vi "visa_close.vi"(2 "err_in":errorcluster, 4 "thcd_visa":refnum<visa-resource-name>) -> (0 "err_out":errorcluster)   [LabVIEW 2019]
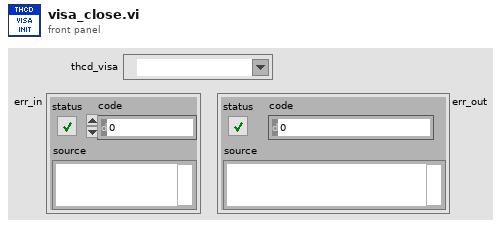
[diagram p1: front panel]
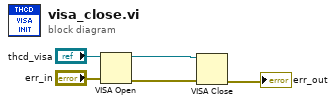
[diagram p0: block diagram]
diagram:
  n1 = VISA Open(error in (no error)="err_in", VISA resource name="thcd_visa") -> (VISA resource name=w1:refnum<visa-resource-name>, error out=w3:errorcluster)  [unwired: 3 in]
  n2 = VISA Close(VISA resource name=w1, error in (no error)=w3) -> (error out=→"err_out":errorcluster)
